vi "Evaluate Part 2.vi"() -> ()   [LabVIEW 2021]
uses:
  Proto/Board.lvclass
panel:
  in  "stop":bool
  out "Waveform Chart":u64(graph)
  out "Load":u64
  in  "Input":string="O....#....\nO.OO#....#\n.....##...\nOO.#O....O\n.O.....O#.\nO.#..O.#.#\n..O..#O..O\n.......O..\n#....###..\n#OO..#...."
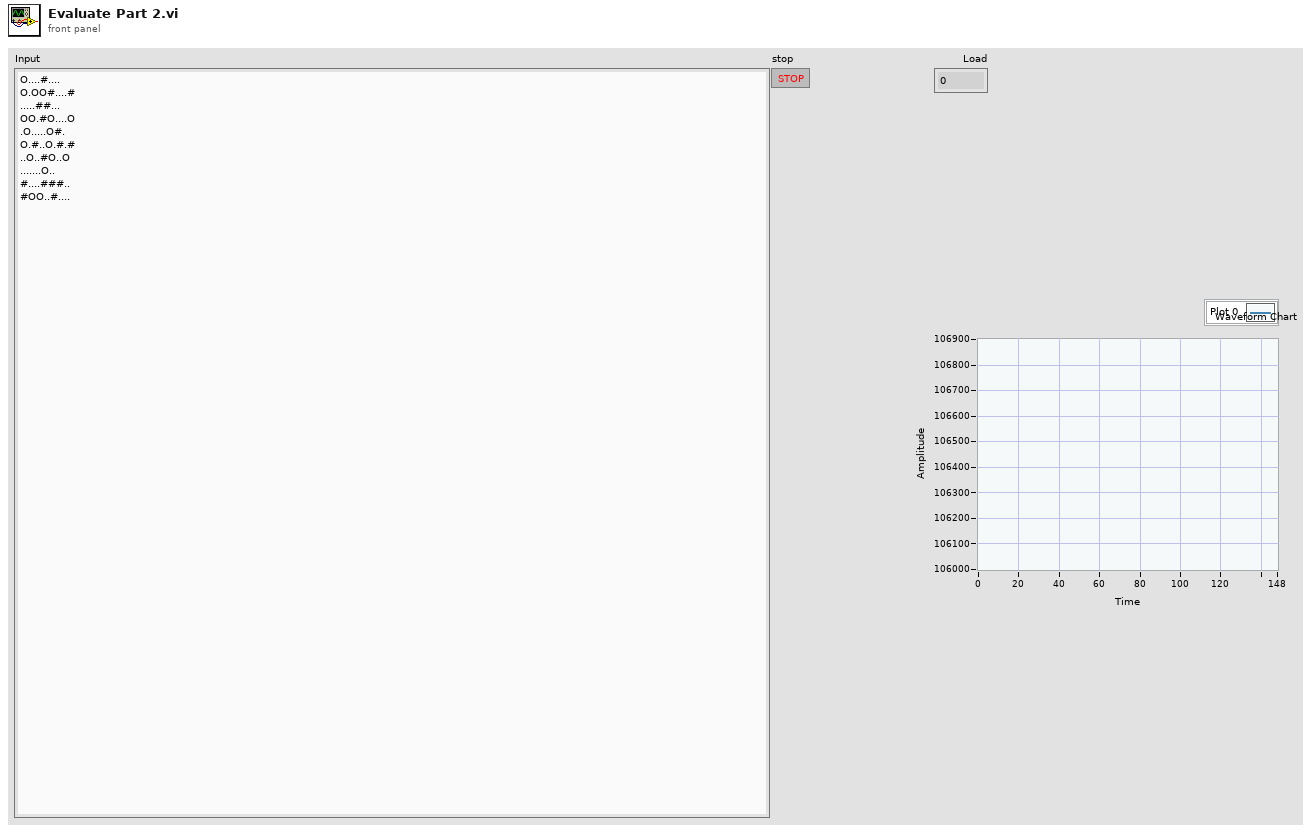
[diagram p1: front panel]
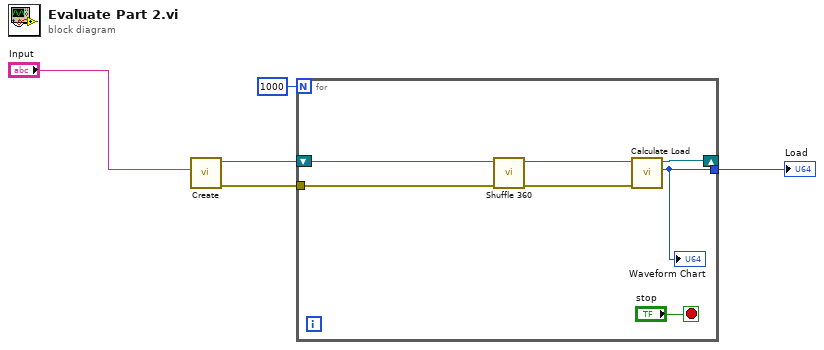
[diagram p0: block diagram]
diagram:
  n1 = call "Create.vi"("Input"="Input") -> ("error out"=w5:errorcluster, "Proto"=w4:refnum<class "Board.lvclass">)  [unwired: 9 in]
  n2 = for {
    N: 1000 -> [_]
    tunnel: w5 -> [w12]
    tunnel: [w7] -> w2
    shift-right: [w8] -> _
    shift-left: w4 -> [w11]
    stop <- "stop" stop-if-true
    n3 = call "Shuffle 360.vi"("error in (no error)"=w12, "Board in"=w11) -> ("error out"=w10:errorcluster, "Board out"=w9:refnum<class "Board.lvclass">)  [unwired: 8 in]
    n4 = call "Calculate Load.vi"("error in (no error)"=w10, "Proto in"=w9) -> ("Load"=w7:u64, "Proto out"=w8:refnum<class "Board.lvclass">)  [unwired: 7 in, 1 out]
    "Waveform Chart" <- w7
  }
  "Load" <- w2
